vi "Maxi Gauge-Test A-D.vi"(0 "VISA-Ressource in":refnum<visa-resource-name>, 1 "Node address":i8=-1 min=-1 max=31 step=1, 3 "Testfunction":u8(ring)=1 items=["A/D Identify", "A/D Sensor"], 5 "Fehler (Eingang)":errorcluster) -> (12 "Channel 1":dbl format="%.3f", 13 "Channel 6":dbl format="%.3f", 14 "VISA-Ressource out":refnum<visa-resource-name>, 15 "Channel 2":dbl format="%.3f", 16 "Channel 3":dbl format="%.3f", 17 "Channel 4":dbl format="%.3f", 18 "Channel 5":dbl format="%.3f", 19 "Fehler (Ausgang)":errorcluster)   [LabVIEW 2012, in "Maxi Gauge.lvlib"]
uses:
  Maxi Gauge.lvlib
panel:
  # "[ V ]"
  # "[ V ]"
  # "[ V ]"
  # "[ V ]"
  # "[ V ]"
  # "[ V ]"
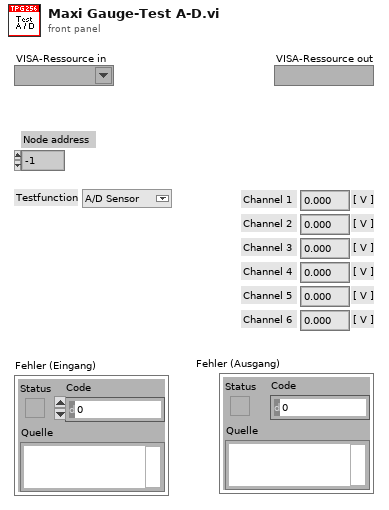
[diagram p1: front panel]
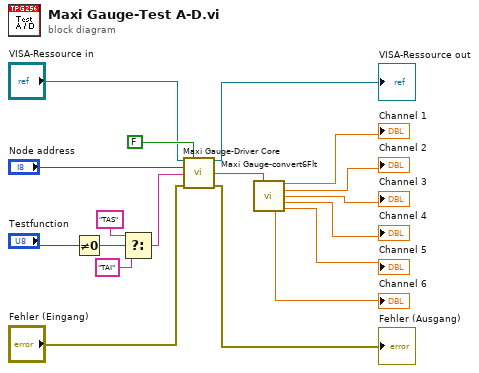
[diagram p0: block diagram]
diagram:
  n1 = Not Equal To 0?(x="Testfunction") -> (x != 0?=w8:bool)
  n2 = Select(t="TAS", s=w8, f="TAI") -> (s? t:f=w5:string)
  n3 = call "Maxi Gauge-Driver Core.vi"("VISA-Ressource in"="VISA-Ressource in", "Write/Read"=FALSE, "Node address"="Node address", "Command"=w5, "Fehler (Eingang)"="Fehler (Eingang)") -> ("VISA-Ressource out"=→"VISA-Ressource out":refnum<visa-resource-name>, "String Out"=w9:string, "Fehler (Ausgang)"=→"Fehler (Ausgang)":errorcluster)  [unwired: 8 in]
  n4 = call "Maxi Gauge-convert6Flt.vi"("String in"=w9) -> ("Fract1 out"=→"Channel 1":dbl, "Fract2 out"=→"Channel 2":dbl, "Fract3 out"=→"Channel 3":dbl, "Fract4 out"=→"Channel 4":dbl, "Fract6 out"=→"Channel 6":dbl, "Fract5 out"=→"Channel 5":dbl)  [unwired: 9 in]
